vi "Add Analog Replay.vi"(8 "error in (no error)":errorcluster, 9 "Analog Replay Data Options":T2={"Selected File"=path "", "Group"="", "Channel"="", "DataPlugin"="", "ReverseData"=FALSE, "FPGA memory size"=enum."16,384", "CycleAngle?"=enum."Crank angle", "Data Selection Method"=enum."Manual", "File start offset"=1, "Samples"=1, "Missing teeth location (degrees)"=1.0} {"Missing teeth location (degrees)" min=0.0; "Samples" min=1; "File start offset" min=0}, 10 "Analog Replay Settings":T1={"Name"="", "RIO Device Address"="", "DAC bipolar range (V)"=0.0001, "Voltage below min speed"=1.0, "Min speed (RPM)"=1.0, "Voltage at min speed"=1.0, "Max speed (RPM)"=1.0, "Voltage at max speed"=1.0, "ReverseNegate"=FALSE, "VOverride"=FALSE} {"Voltage at max speed" min=0.0 max=10.0; "Max speed (RPM)" min=0.0 max=10.0; "Voltage at min speed" min=1.0; "Min speed (RPM)" min=0.0 max=10.0; "Voltage below min speed" min=0.0; "DAC bipolar range (V)" min=0.0 max=10.0}, 11 "APU in":refnum<k24>) -> (0 "error out":errorcluster, 2 "Analog Replay":refnum<k24>, 3 "APU out":refnum<k24>)   [LabVIEW 2015, in "Engine Simulation Toolkit Scripting API.lvlib"]
uses:
  Engine Simulation Toolkit Scripting API.lvlib
  NationalInstruments.VeriStand.SystemDefinitionAPI
  Analog Replay Data Options.ctl
  System Explorer/FPGA Mem Size.ctl
  System Explorer/Position Reference.ctl
  System Explorer/Data Replay Data Selection Method.ctl
  Analog Replay Settings.ctl
  Shared/Constants and GUIDs.vi
  <vilib>/NI Veristand/Custom Device Tools/Custom Device Utility Library/NI VeriStand - Search for Item by GUID.vi
  System Explorer/Engine Simulation Toolkit System Explorer.lvlib
  <vilib>/NI VeriStand/Custom Device API/Custom Device API.lvlib
  <vilib>/NI VeriStand/Custom Device Tools/Custom Device Utility Library/Custom Device Utility Library.lvlib
  Shared/Engine Simulation Toolkit Shared.lvlib
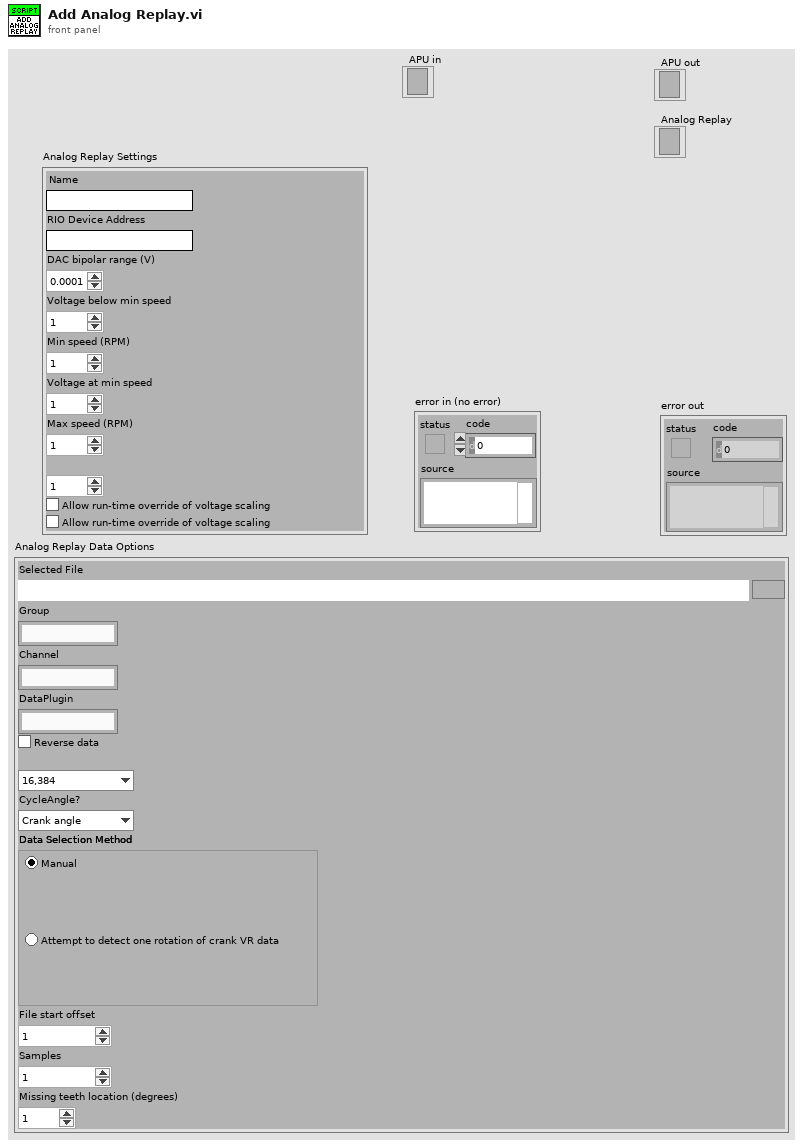
[diagram p1: front panel]
types:
  T1 = typedef "Engine Simulation Toolkit Scripting API.lvlib/Analog Replay Settings.ctl" = cluster{"Name":string, "RIO Device Address":string, "DAC bipolar range (V)":dbl, "Voltage below min speed":dbl, "Min speed (RPM)":dbl, "Voltage at min speed":dbl, "Max speed (RPM)":dbl, "Voltage at max speed":dbl, "ReverseNegate":bool, "VOverride":bool}
  T2 = typedef "Engine Simulation Toolkit Scripting API.lvlib/Analog Replay Data Options.ctl" = cluster{"Selected File":path, "Group":string, "Channel":string, "DataPlugin":string, "ReverseData":bool, "FPGA memory size":T3, "CycleAngle?":T4, "Data Selection Method":T5, "File start offset":i32, "Samples":i32, "Missing teeth location (degrees)":dbl}
  T3 = typedef "Engine Simulation Toolkit System Explorer.lvlib/FPGA Mem Size.ctl" = enum16{"65,536", "32,768", "16,384", "8,192", "4,096", "2,048", "1,024"}
  T4 = typedef "Engine Simulation Toolkit System Explorer.lvlib/Position Reference.ctl" = enum16{"Crank angle", "Cycle angle"}
  T5 = typedef "Engine Simulation Toolkit System Explorer.lvlib/Data Replay Data Selection Method.ctl" = enum32{"Manual", "AutoVRCrank"}
  T6 = typedef "Custom Device API.lvlib/Custom Device Item Ref.ctl" = u64
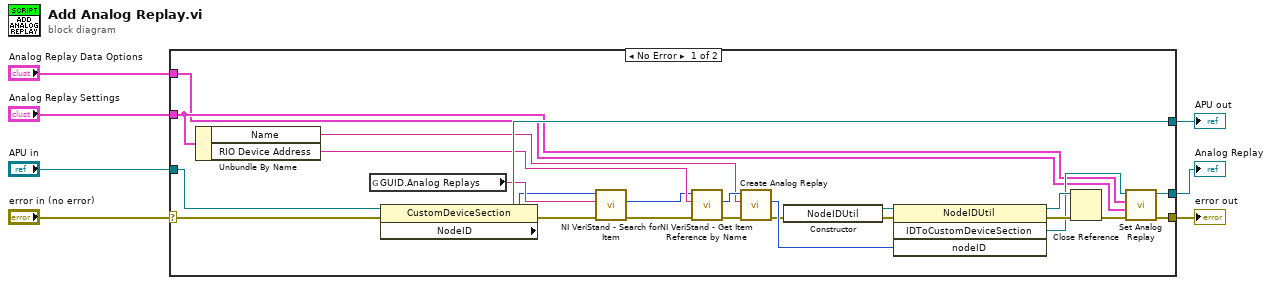
[diagram p0: block diagram]
diagram:
  n1 = case shown="No Error" "error in (no error)" {
    selector: "error in (no error)" -> [w31 w33]
    tunnel: [w17 w33] -> w7
    tunnel: "Analog Replay Data Options" -> [w13 _]
    tunnel: "APU in" -> [w26 w32]
    tunnel: "Analog Replay Settings" -> [w14 _]
    tunnel: [w25 w32] -> w2
    tunnel: [w15 _] -> w1
    frame No Error {
      n2 = Unbundle By Name(w14) -> ("Name"=w22:string, "RIO Device Address"=w23:string)
      n3 = global read "Constants and GUIDs.vi" "GUID.Analog Replays"() -> (w12:string)
      n4 = property class="CustomDeviceSection"(reference=w26, error in=w31) -> (reference out=w25:refnum<k24>, error out=w9:errorcluster, "NodeID"=w11:u64)
      n5 = call-poly <vilib>:"NI VeriStand - Search for Item.vi"("error in"=w9, "Item GUID"=w12, "Section Ref in"=w11) -> ("error out"=w8:errorcluster, "Item Ref"=w10:T6)  [unwired: 5 in, 2 out]
      n6 = call <vilib>:"NI VeriStand - Get Item Reference by Name.vi"("error in (no error)"=w8, "Item Name"=w23, "Parent Ref in"=w10) -> ("error out"=w21:errorcluster, "Item Ref"=w24:T6)  [unwired: 5 in, 2 out]
      n7 = call "Create Analog Replay.vi"("error in (no error)"=w21, "analog replay name"=w22, "Section Ptr"=w24) -> ("error out"=w19:errorcluster, "Analog replay ref"=w20:T6)  [unwired: 6 in, 1 out]
      n8 = constructor class="NodeIDUtil"(error in=w19) -> (reference out=w29:refnum<k24>, error out=w30:errorcluster)  [unwired: 2 in, 1 out]
      n9 = invoke class="NodeIDUtil" method="IDToCustomDeviceSection"(reference=w29, error in=w30, "nodeID"=w20) -> (reference out=w28:refnum<k24>, error out=w27:errorcluster, "IDToCustomDeviceSection"=w16:refnum<k24>)  [unwired: 1 in, 1 out]
      n10 = Close Reference(reference=w28, error in (no error)=w27) -> (error out=w18:errorcluster)
      n11 = call "Set Analog Replay.vi"("error in (no error)"=w18, "Analog Replay Data Options"=w13, "Analog Replay Settings"=w14, "Analog Replay in"=w16) -> ("error out"=w17:errorcluster, "Analog Replay out"=w15:refnum<k24>)  [unwired: 6 in]
    }
    frame Error {
    }
  }
  "error out" <- w7
  "APU out" <- w2
  "Analog Replay" <- w1
